vi "sensor de flama.vi"() -> ()   [LabVIEW 2016]
uses:
  <vilib>/LabVIEW Interface for Arduino/Type Defs/Board Type.ctl
  <vilib>/LabVIEW Interface for Arduino/Type Defs/Connection Type.ctl
  <vilib>/LabVIEW Interface for Arduino/LabVIEW Interface for Arduino.lvlib
panel:
  in  "stop":bool
  out "Digita;":bool
  out "Analog":dbl(knob) scale=0.0..10.0
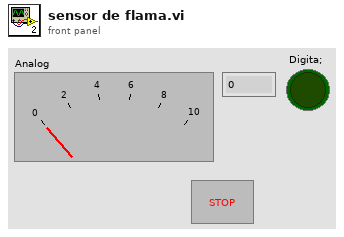
[diagram p1: front panel]
types:
  T1 = typedef "LabVIEW Interface for Arduino.lvlib/Connection Type.ctl" = enum8{"USB / Serial", "XBEE", "BlueSmirf (Bluetooth)"}
  T2 = typedef "LabVIEW Interface for Arduino.lvlib/Board Type.ctl" = enum16{"Uno", "Dimuelanove w/Atmega 328", "Mega 2560"}
  T3 = typedef "LabVIEW Interface for Arduino.lvlib/Arduino Resource.ctl" = cluster{"VISA resource":refnum<visa-resource-name>, "Board Type":T2, "Connection Type":enum8{"USB / Serial"}, "Bytes Per Packet (15)":u8}
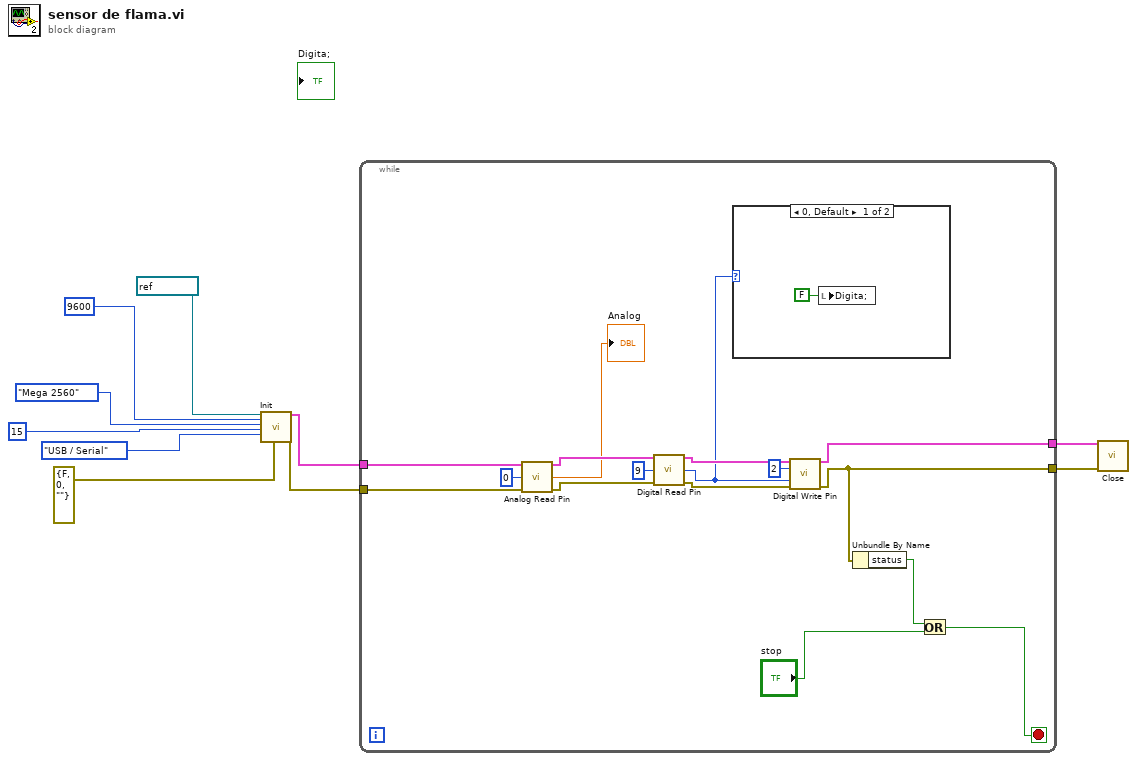
[diagram p0: block diagram]
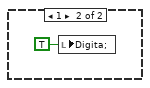
[diagram p2: hidden frame]
diagram:
  n1 = call <vilib>:"Init.vi"("VISA resource"=refnum<visa-resource-name> "COM6", "Baud Rate (115200)"=u32 9600, "Board Type (Uno)"=Board_Type."Mega 2560", "Bytes Per Packet (15)"=u32 15, "Connection Type (USB/Serial)"=Connection_Type."USB / Serial", "error in"=errorcluster {"status"=FALSE, "code"=0, "source"=""}) -> ("Arduino Resource"=w4:T3, "error out"=w3:errorcluster)  [unwired: 12 in]
  n2 = while {
    tunnel: w4 -> [w26]
    tunnel: w3 -> [w24]
    tunnel: [w20] -> w2
    tunnel: [w19] -> w1
    stop <- w18 stop-if-true
    n3 = call <vilib>:"Analog Read Pin.vi"("Arduino Resource"=w26, "Analog Input Pin (0)"=u8 0, "error in"=w24) -> ("Arduino Resource"=w25:T3, "Voltage"=→"Analog":dbl, "error out"=w23:errorcluster)  [unwired: 10 in]
    n4 = call <vilib>:"Digital Read Pin.vi"("Arduino Resource"=w25, "Digital I/O Pin (0)"=u8 9, "error in"=w23) -> ("Arduino Resource"=w22:T3, "Value"=w14:u8, "error out"=w21:errorcluster)  [unwired: 10 in]
    n5 = case shown="0, Default" w14 {
      frame 0, Default {
        n6 = local write "Digita;"(FALSE ("Digita;")) -> ()
      }
      frame 1 {
        n7 = local write "Digita;"(TRUE ("Digita;")) -> ()
      }
    }
    n8 = call <vilib>:"Digital Write Pin.vi"("Arduino Resource"=w22, "Digital I/O Pin (0)"=u8 2, "Value (0)"=w14, "error in"=w21) -> ("Arduino Resource"=w20:T3, "error out"=w19:errorcluster)  [unwired: 10 in]
    n9 = Unbundle By Name(w19) -> ("status"=w17:bool)
    n10 = Or(x=w17, y="stop") -> (x .or. y?=w18:bool)
  }
  n11 = call <vilib>:"Close.vi"("Arduino Resource"=w2, "error in"=w1) -> ()  [unwired: 13 in, 1 out]
